vi "SubModule Config.vi"(6 "Status":bool, 8 "error in (no error)":errorcluster, 9 "Cycles":i32, 10 "Name":string, 11 "Camera in":refnum<class "Camera.lvclass">) -> (0 "error out":errorcluster, 3 "Camera out":refnum<class "Camera.lvclass">)   [LabVIEW 2021, in "Camera.lvclass"]
uses:
  Camera.lvclass
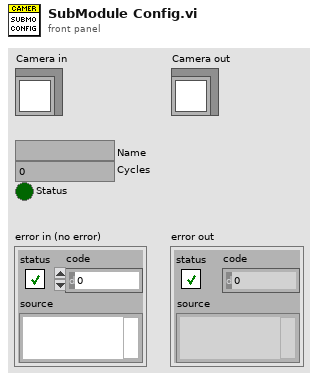
[diagram p1: front panel]
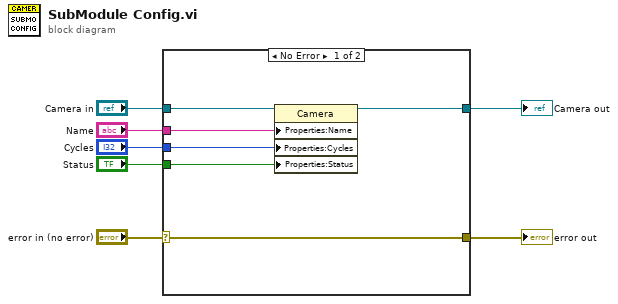
[diagram p0: block diagram]
diagram:
  n1 = case shown="No Error" "error in (no error)" {
    selector: "error in (no error)" -> [w12 w15]
    tunnel: [w12 w15] -> w6
    tunnel: [w11 w14] -> w4
    tunnel: "Camera in" -> [w13 w14]
    tunnel: "Name" -> [w10 _]
    tunnel: "Cycles" -> [w9 _]
    tunnel: "Status" -> [w8 _]
    frame No Error {
      n2 = property class="Camera"(reference=w13, "Properties:Name"=w10, "Properties:Cycles"=w9, "Properties:Status"=w8) -> (reference out=w11:refnum<class "Camera.lvclass">)  [unwired: 1 in, 1 out]
    }
    frame Error {
    }
  }
  "error out" <- w6
  "Camera out" <- w4
